vi "Tree Set Active Tree.vi"(8 "error in (no error)":errorcluster, 9 "Tree in":refnum<data-value>, 11 "Tree DVR in":refnum<data-value>) -> (0 "error out":errorcluster, 1 "Tree out":refnum<data-value>, 3 "Tree DVR out":refnum<data-value>)   [LabVIEW 2010, in "MDSplus.lvlib"]
doc: "Set the passed tree as the active one."
uses:
  <vilib>/MDSplus/Library/MDSplus.lvlib
  <vilib>/MDSplus/Classes/Data_Class/Data.lvclass
  <vilib>/MDSplus/Classes/Tree_Class/Tree.lvclass
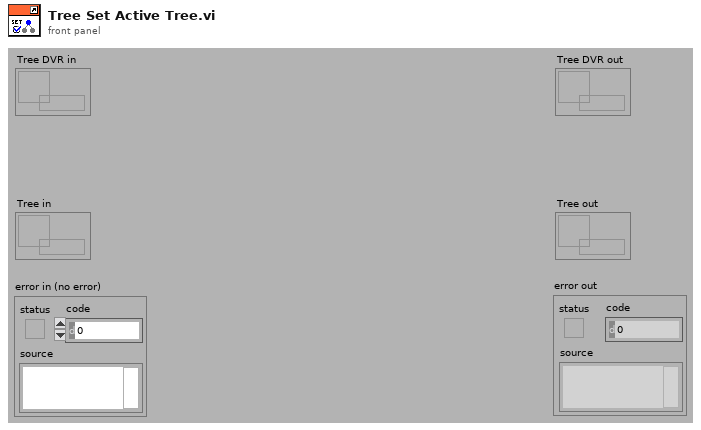
[diagram p1: front panel]
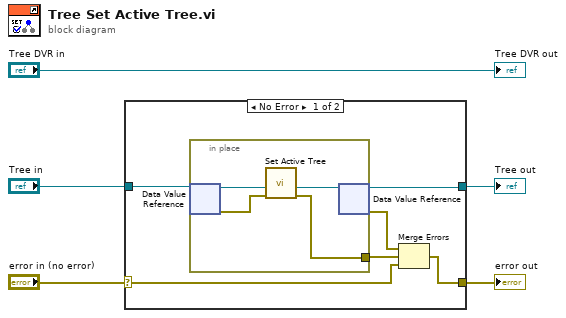
[diagram p0: block diagram]
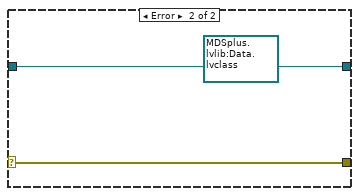
[diagram p2: hidden frame]
diagram:
  n1 = case shown="No Error" "error in (no error)" {
    selector: "error in (no error)" -> [w11 w18]
    tunnel: [w10 w18] -> w3
    tunnel: "Tree in" -> [w9 w16]
    tunnel: [w8 w16] -> w2
    frame No Error {
      n2 = in-place {
        in-place-border: [w12] -> w6
        n3 = in-place-dvr #1(w9) -> (w14:refnum<class "Tree.lvclass">, w15:errorcluster)
        n4 = call <vilib>:"Set Active Tree.vi"("error in (no error)"=w15, "Tree to set in"=w14) -> ("error out"=w12:errorcluster, "Tree set out"=w13:refnum<class "Tree.lvclass">)  [unwired: 7 in, 1 out]
        n5 = in-place-dvr #1(w13) -> (w8:refnum<data-value>, w7:errorcluster)
      }
      n6 = Merge Errors(w7, w6, w11) -> (w10:errorcluster)
    }
    frame Error {
      w17 = refnum<data-value> refnum ("TreeNode DVR out")
    }
  }
  "error out" <- w3
  "Tree out" <- w2
  "Tree DVR out" <- "Tree DVR in"
